vi "QrCodeBuild-Zxing.vi"(3 "ErrorCorrectLevel":i32(ring)=1 items=["L", "M", "Q", "H"], 4 "Scale":u8=4, 5 "Text":string="31S5106            W84B9L004        20180419SBDCNMR-JE-70B                      0001") -> (1 "out Array":bool[][](array[boolean]))   [LabVIEW 2018]
uses:
  zxing.dll
  <vilib>/picture/picture.llb/Draw 1-Bit Pixmap.vi
panel:
  out "二维图片":picture
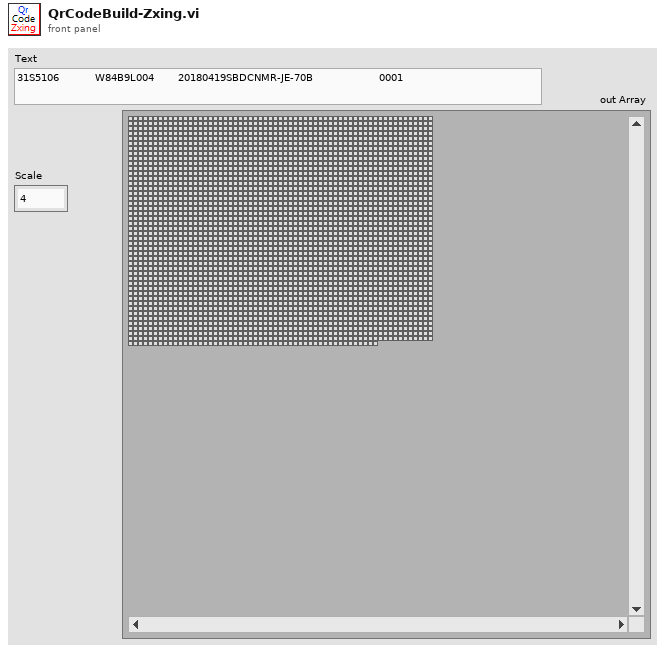
[diagram p1: front panel]
types:
  T1 = typedef "imagedata.ctl" = cluster{"image type":i32, "image depth":i32, "image":u8[], "mask":u8[], "colors":u32[], "Rectangle":cluster{"left":i16, "top":i16, "right":i16, "bottom":i16}}
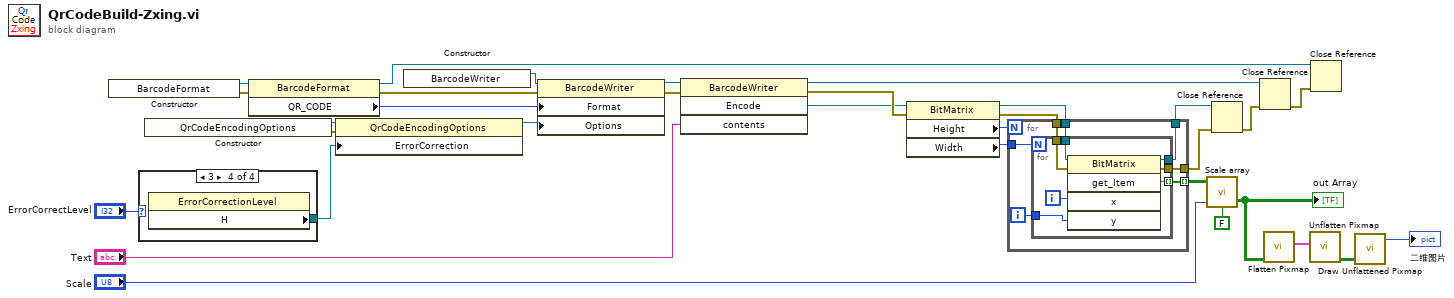
[diagram p0: block diagram]
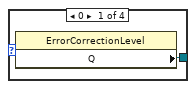
[diagram p2: hidden frame]
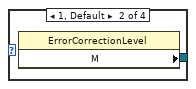
[diagram p3: hidden frame]
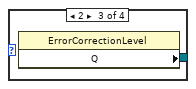
[diagram p4: hidden frame]
diagram:
  n1 = constructor class="BarcodeFormat"() -> (reference out=w31:refnum<k24>, error out=w32:errorcluster)  [unwired: 3 in, 1 out]
  n2 = case shown="3" "ErrorCorrectLevel" {
    tunnel: [w33 w34 w35 w36] -> w28
    frame 0 {
      n3 = property class="ErrorCorrectionLevel"() -> ("Q"=w33:refnum<k24>)  [unwired: 2 in, 2 out]
    }
    frame 1, Default {
      n4 = property class="ErrorCorrectionLevel"() -> ("M"=w34:refnum<k24>)  [unwired: 2 in, 2 out]
    }
    frame 2 {
      n5 = property class="ErrorCorrectionLevel"() -> ("Q"=w35:refnum<k24>)  [unwired: 2 in, 2 out]
    }
    frame 3 {
      n6 = property class="ErrorCorrectionLevel"() -> ("H"=w36:refnum<k24>)  [unwired: 2 in, 2 out]
    }
  }
  n7 = constructor class="QrCodeEncodingOptions"() -> (reference out=w23:refnum<k24>, error out=w11:errorcluster)  [unwired: 3 in, 1 out]
  n8 = property class="BarcodeFormat"(reference=w31, error in=w32) -> (reference out=w7:refnum<k24>, error out=w15:errorcluster, "QR_CODE"=w30:i32)
  n9 = property on="属性节点" class="QrCodeEncodingOptions"(reference=w23, error in=w11, "ErrorCorrection"=w28) -> (reference out=w29:refnum<k24>)  [unwired: 1 out]
  n10 = constructor class="BarcodeWriter"() -> (reference out=w24:refnum<k24>)  [unwired: 3 in, 2 out]
  n11 = property class="BarcodeWriter"(reference=w24, error in=w15, "Format"=w30, "Options"=w29) -> (reference out=w26:refnum<k24>, error out=w27:errorcluster)
  n12 = invoke class="BarcodeWriter" method="Encode"(reference=w26, error in=w27, "contents"="Text") -> (reference out=w17:refnum<k24>, error out=w14:errorcluster, "Encode"=w6:refnum<k24>)  [unwired: 1 in, 1 out]
  n13 = property class="BitMatrix"(reference=w6, error in=w14) -> (reference out=w13:refnum<k24>, error out=w12:errorcluster, "Height"=w22:i32, "Width"=w21:i32)
  n14 = for {
    N: w22 -> [_]
    tunnel: w21 -> [w43]
    tunnel: [w41] -> w2 mode=indexing
    tunnel: [w40] -> w9
    tunnel: [w39] -> w10
    tunnel: w13 -> [w38]
    tunnel: w12 -> [w37]
    i -> [w42]
    n15 = for {
      N: w43 -> [_]
      tunnel: w42 -> [w49]
      tunnel: [w48] -> w41 mode=indexing
      tunnel: [w47] -> w40
      tunnel: [w46] -> w39
      tunnel: w38 -> [w45]
      tunnel: w37 -> [w44]
      i -> [w50]
      n16 = invoke class="BitMatrix" method="get_Item"(reference=w45, error in=w44, "x"=w50, "y"=w49) -> (reference out=w47:refnum<k24>, error out=w46:errorcluster, "get_Item"=w48:bool)  [unwired: 1 in, 2 out]
    }
  }
  n17 = call "Scale array.vi"("有边缘？"=FALSE, "Scale"="Scale", "in Array"=w2) -> ("out Array"=w1:bool[][])  [unwired: 1 in, 1 out]
  "out Array" <- w1
  n18 = Close Reference(reference=w9, error in (no error)=w10) -> (error out=w16:errorcluster)
  n19 = Close Reference(reference=w17, error in (no error)=w16) -> (error out=w8:errorcluster)
  n20 = call <vilib>:"Flatten Pixmap.vi"("1-bit pixmap"=w1) -> ("image data"=w5:T1)  [unwired: 10 in]
  n21 = call <vilib>:"Unflatten Pixmap.vi"("image data"=w5) -> ("1-bit pixmap"=w3:bool[][])  [unwired: 4 in, 6 out]
  n22 = Close Reference(reference=w7, error in (no error)=w8) -> ()  [unwired: 1 out]
  n23 = call-poly <vilib>:"Draw Unflattened Pixmap.vi"("data"=w3) -> ("new picture"=→"二维图片":picture)  [unwired: 8 in]
